vi "SpreadsheetRead.vi"() -> ()   [LabVIEW 2014]
uses:
  <vilib>/Utility/file.llb/Read From Spreadsheet File (I64).vi
panel:
  out "XY Graph":cluster{"X":dbl, "Y":dbl}[](graph)
  in  "file path (dialog if empty)":path
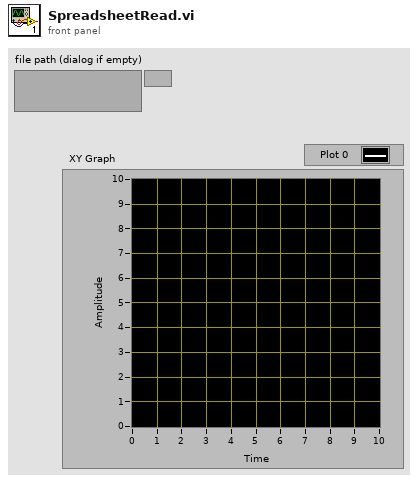
[diagram p1: front panel]
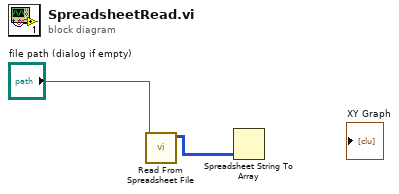
[diagram p0: block diagram]
diagram:
  n1 = call-poly <vilib>:"Read From Spreadsheet File.vi"("file path (dialog if empty)"="file path (dialog if empty)") -> ("all rows"=w1:i64[][])  [unwired: 6 in, 4 out]
  n2 = Spreadsheet String To Array(array type (2D Dbl)=w1) -> ()  [unwired: 3 in, 1 out]
